vi "MicroRowClicked.vi"(4 "UiDefinition":T1, 5 "Event Data":cluster{"sender":refnum<k24>, "e":refnum<k24>}, 6 "Control Ref":refnum<k24>, 7 "Event Common Data":T2) -> ()   [LabVIEW 2020]
uses:
  C:/Users/User/Desktop/Automation/CurrentVersion/LabviewDXFViewer/bin/Release/LabviewDXFViewer.exe
  CurrentVersion/LabviewDXFViewer/bin/Release/LabviewDXFViewer.exe
  CurrentVersion/AutomatedProbing/UIReferences.ctl
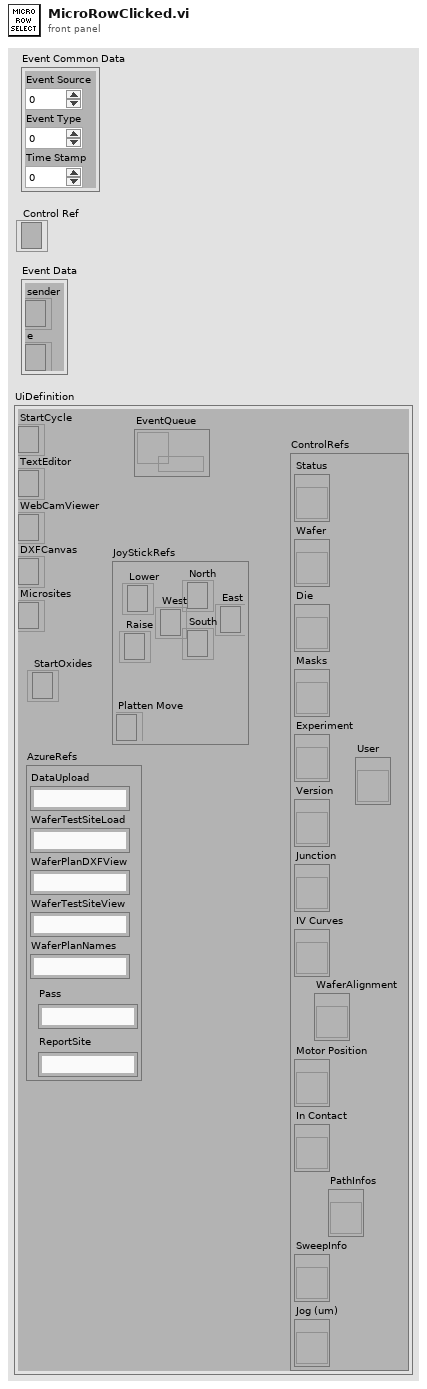
[diagram p1: front panel]
types:
  T1 = typedef "UIReferences.ctl" = cluster{"StartCycle":refnum<k24>, "TextEditor":refnum<k24>, "WebCamViewer":refnum<k24>, "DXFCanvas":refnum<k24>, "Microsites":refnum<k24>, "JoyStickRefs":cluster{"North":refnum<k24>, "Lower":refnum<k24>, "Raise":refnum<k24>, "Platten Move":refnum<k24>, "West":refnum<k24>, "East":refnum<k24>, "South":refnum<k24>}, "AzureRefs":cluster{"DataUpload":string, "WaferTestSiteLoad":string, "WaferPlanDXFView":string, "WaferTestSiteView":string, "WaferPlanNames":string, "Pass":string, "ReportSite":string}, "ControlRefs":cluster{"Status":refnum<vi>, "Wafer":refnum<vi>, "Die":refnum<vi>, "Masks":refnum<vi>, "Experiment":refnum<vi>, "Version":refnum<vi>, "Junction":refnum<vi>, "IV Curves":refnum<vi>, "Motor Position":refnum<vi>, "In Contact":refnum<vi>, "SweepInfo":refnum<vi>, "Jog (um)":refnum<vi>, "PathInfos":refnum<vi>, "User":refnum<vi>, "WaferAlignment":refnum<vi>}, "EventQueue":refnum<queue>, "StartOxides":refnum<k24>}
  T2 = cluster{"Event Source":i32, "Event Type":u32, "Time Stamp":u32}
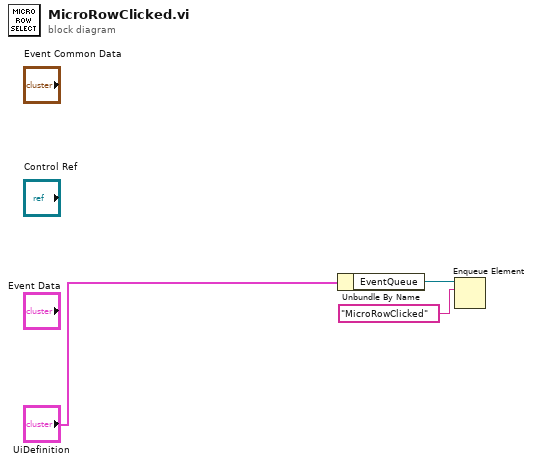
[diagram p0: block diagram]
diagram:
  n1 = Unbundle By Name("UiDefinition") -> ("EventQueue"=w3:refnum<queue>)
  n2 = Enqueue Element(queue=w3, element="MicroRowClicked") -> ()  [unwired: 2 in, 3 out]
